vi "phan_songsong.vi"() -> ()   [LabVIEW 2019]
uses:
  <vilib>/Platform/TimedLoop/XDataNode/timing_clust.ctl
  <vilib>/Platform/TimedLoop/XDataNode/nitl_modes.ctl
  <vilib>/Platform/TimedLoop/XDataNode/wakeup.ctl
  <vilib>/platform/TimedLoop/XDataNode/XDataNode.xnode
  <vilib>/Platform/TimedLoop/XDataNode/XDNodeRunTimeDep.lvlib
  <vilib>/ptbypt/NI_PtbyPt.lvlib
panel:
  out "S":dbl
  out "yo":dbl
  out "xo":dbl
  out "yb":dbl
  out "xb":dbl
  out "ya":dbl
  out "xa":dbl
  out "c":dbl
  out "y_o":dbl
  out "x_o":dbl
  in  "vantocgocmax":dbl=1.5
  in  "vantocmax":dbl=0.5
  out "phi_ph":dbl
  out "wdk":dbl
  out "phi_sp":dbl
  in  "Kiw":dbl
  in  "Kpw":dbl=3.0
  in  "Kdw":dbl
  out "Vxdk":dbl
  out "Vydk":dbl
  in  "Kdv3":dbl
  in  "Kiv3":dbl=28.5
  in  "Kpv3":dbl=0.7
  in  "Kdv2":dbl
  in  "Kiv2":dbl=28.5
  in  "Kpv2":dbl=0.7
  out "Ts":dbl=10.0
  out "TOA DO 2":dbl[][](array[numeric])
  out "sailechxy":cluster{"e_phi":dbl, "e_x":dbl, "e_y":dbl}(graph)
  in  "Kdxy":dbl
  in  "Kixy":dbl
  in  "Kpxy":dbl=4.0
  in  "?":enum32{"DUONG 2", "DUONGTRON", "NHAP DIEM"}(tab)
  in  "xstart":dbl format="%#_13g"
  in  "xend":dbl=2.0
  in  "time2":dbl=10.0
  in  "R":dbl=0.6
  in  "phi_end":dbl=15.71
  in  "phi_start":dbl=3.14159 format="%#_13g"
  out "time":dbl
  in  "y2":dbl
  in  "x1":dbl
  in  "x2":dbl
  in  "x3":dbl
  in  "y3":dbl
  in  "y1":dbl
  in  "x4":dbl
  in  "y4":dbl
  out "time":dbl
  out "buoc":dbl
  out "V_ph":dbl
  out "w_ph3":dbl
  out "w_ph2":dbl
  out "w_ph1":dbl
  in  "RESETMAP":bool=TRUE caption="Reset"
  out "duty3":dbl
  out "duty2":dbl
  out "duty1":dbl
  in  "RESET":bool
  out "Y_sp":dbl
  out "X_sp":dbl
  out "Y_ph":dbl
  out "X_ph":dbl
  out "Map":cluster{"Y":dbl[], "Y":dbl[]}[](graph)
  out "V3_sp":dbl
  out "V3_ph":dbl
  out "VAN TOC":T1(graph)
  in  "Kdv1":dbl
  in  "Kiv1":dbl=28.5
  in  "Kpv1":dbl=0.7
  out "V2_ph":dbl
  out "V1_ph":dbl
  out "V2_sp":dbl
  out "V1_sp":dbl
  in  "START":bool
  # "HE THONG"
  # "PID VI TRI"
  # "PID TOC DO"
  # "VI TRI DIEU KHIEN\n(m)"
  # "VI TRI PHAN HOI\n(m)"
  # "Van toc dat"
  # "VAN TOC DIEU KHIEN\n(m/s)"
  # "VAN TOC PHAN HOI\n(m/s)"
  # "DUTY"
  # "TOC DO PHAN HOI (rad/s)"
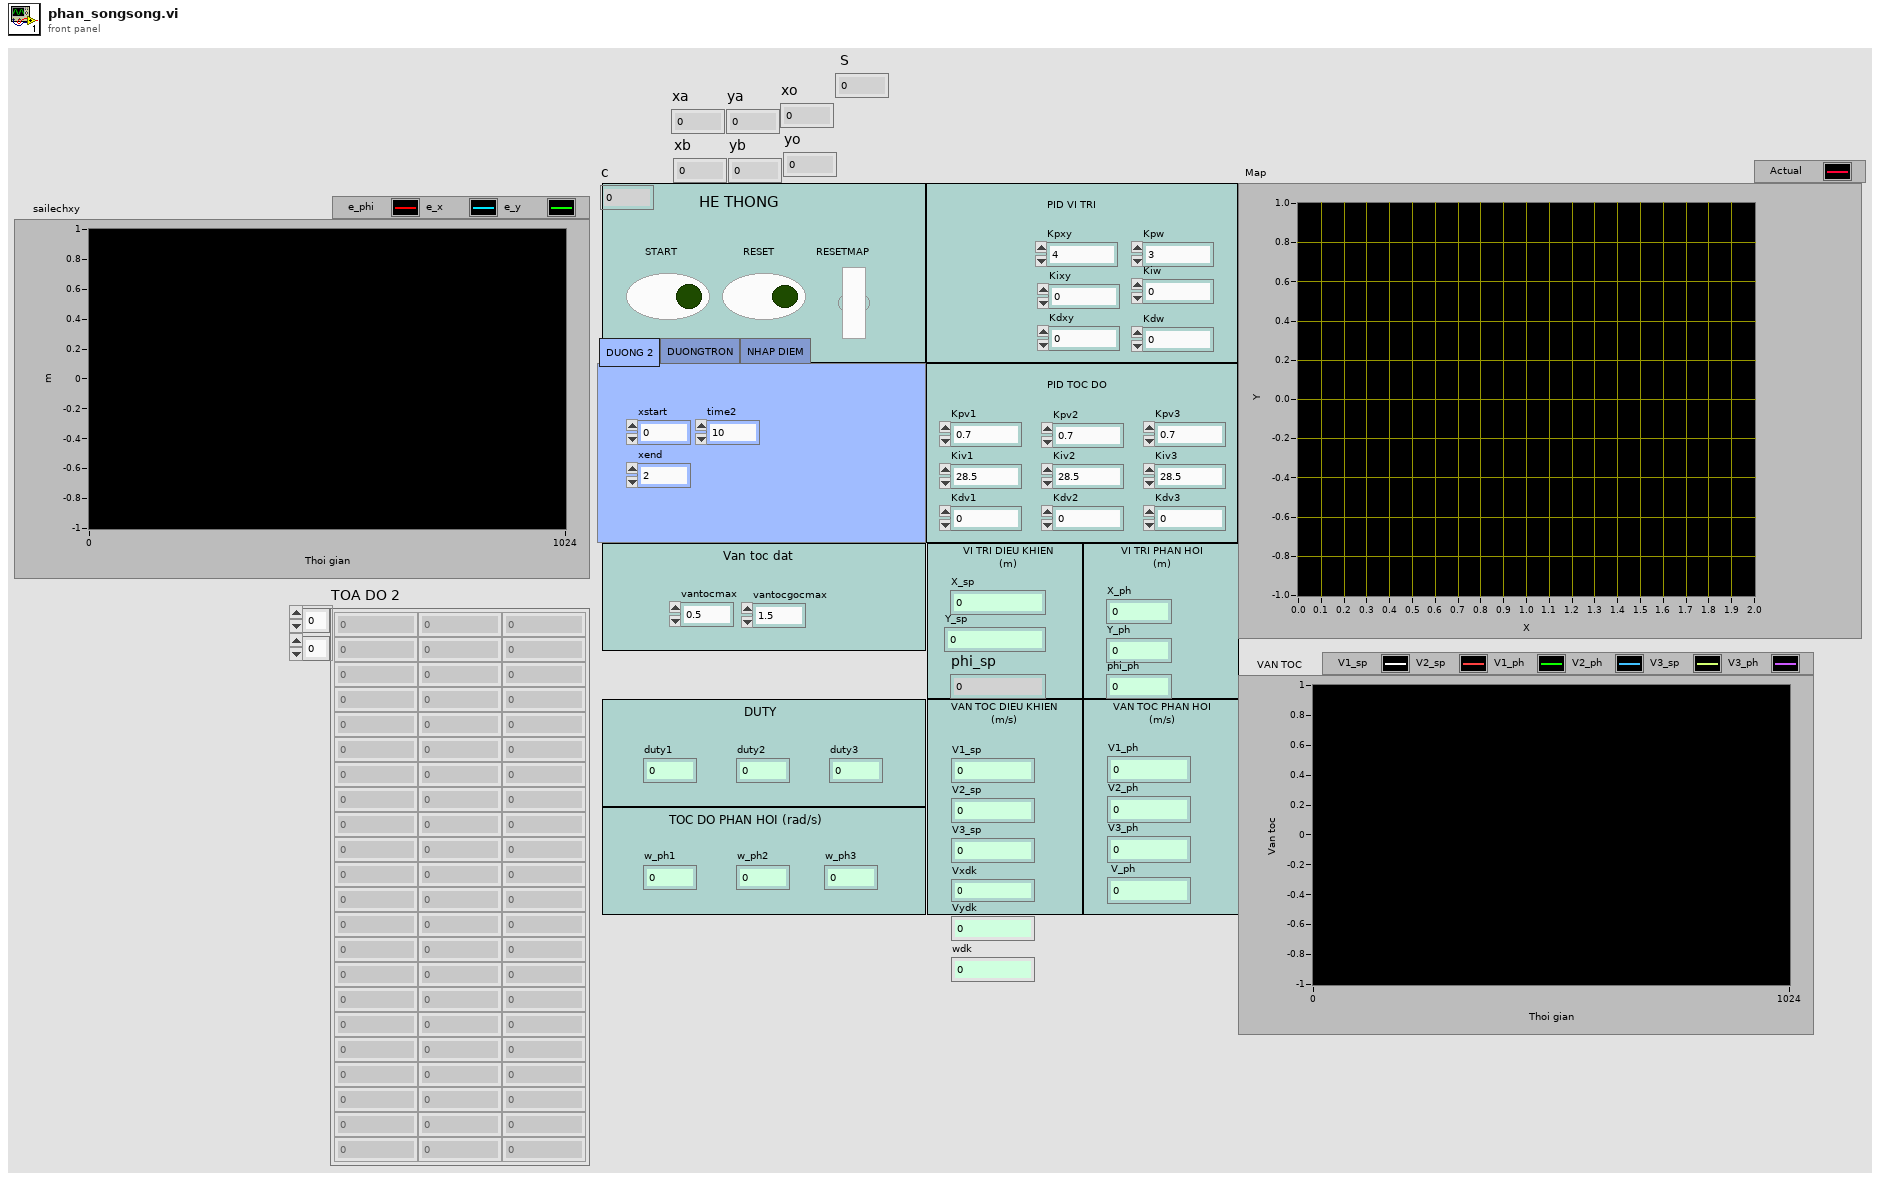
[diagram p1: front panel]
types:
  T1 = cluster{dbl, dbl, "V1_ph":dbl, "V2_ph":dbl, dbl, "V3_ph":dbl}
  T2 = typedef "XDNodeRunTimeDep.lvlib/timing_clust.ctl" = cluster{"Expected End [f-1]":u64, "Actual End [f-1]":u64, "Finished Late? [f-1]":bool, "Expected End [i-1]":u64, "Actual End [i-1]":u64, "Finished Late? [i-1]":bool, "Expected Start [i]":u64, "Actual Start [i]":u64, "Expected Start [f]":u64, "Actual Start [f]":u64, "Source Name":string, "Structure Name":string, "Period":i64, "Deadline":i64, "Offset":i64, "Start":i64, "Priority":i32, "Timeout":i32, "Mode":T3, "Wakeup Reason":T4, "Error":errorcluster, "Source Type":string, "Secondary Source Type":string, "Global End Time":u64, "Global Start Time":u64, "Frame Duration":u64, "Iteration Duration":u64, "Assigned CPU":i32, "I/O Scan Engine Mode":u32}
  T3 = typedef "XDNodeRunTimeDep.lvlib/nitl_modes.ctl" = enum32{"No Change", "Process missed periods, maintain original phase", "Discard missed periods, maintain original phase", "Process missed periods, ignore original phase", "Discard missed periods, ignore original phase"}
  T4 = typedef "XDNodeRunTimeDep.lvlib/wakeup.ctl" = enum32{"Normal", "Aborted", "Asynchronous wakeup", "Timing source error", "Timed loop error", "Timeout"}
  T5 = cluster{"V1_sp":dbl, "V_ph1":dbl, "V2_sp":dbl, "V_ph2":dbl, "V3_sp":dbl, "V_ph3":dbl}
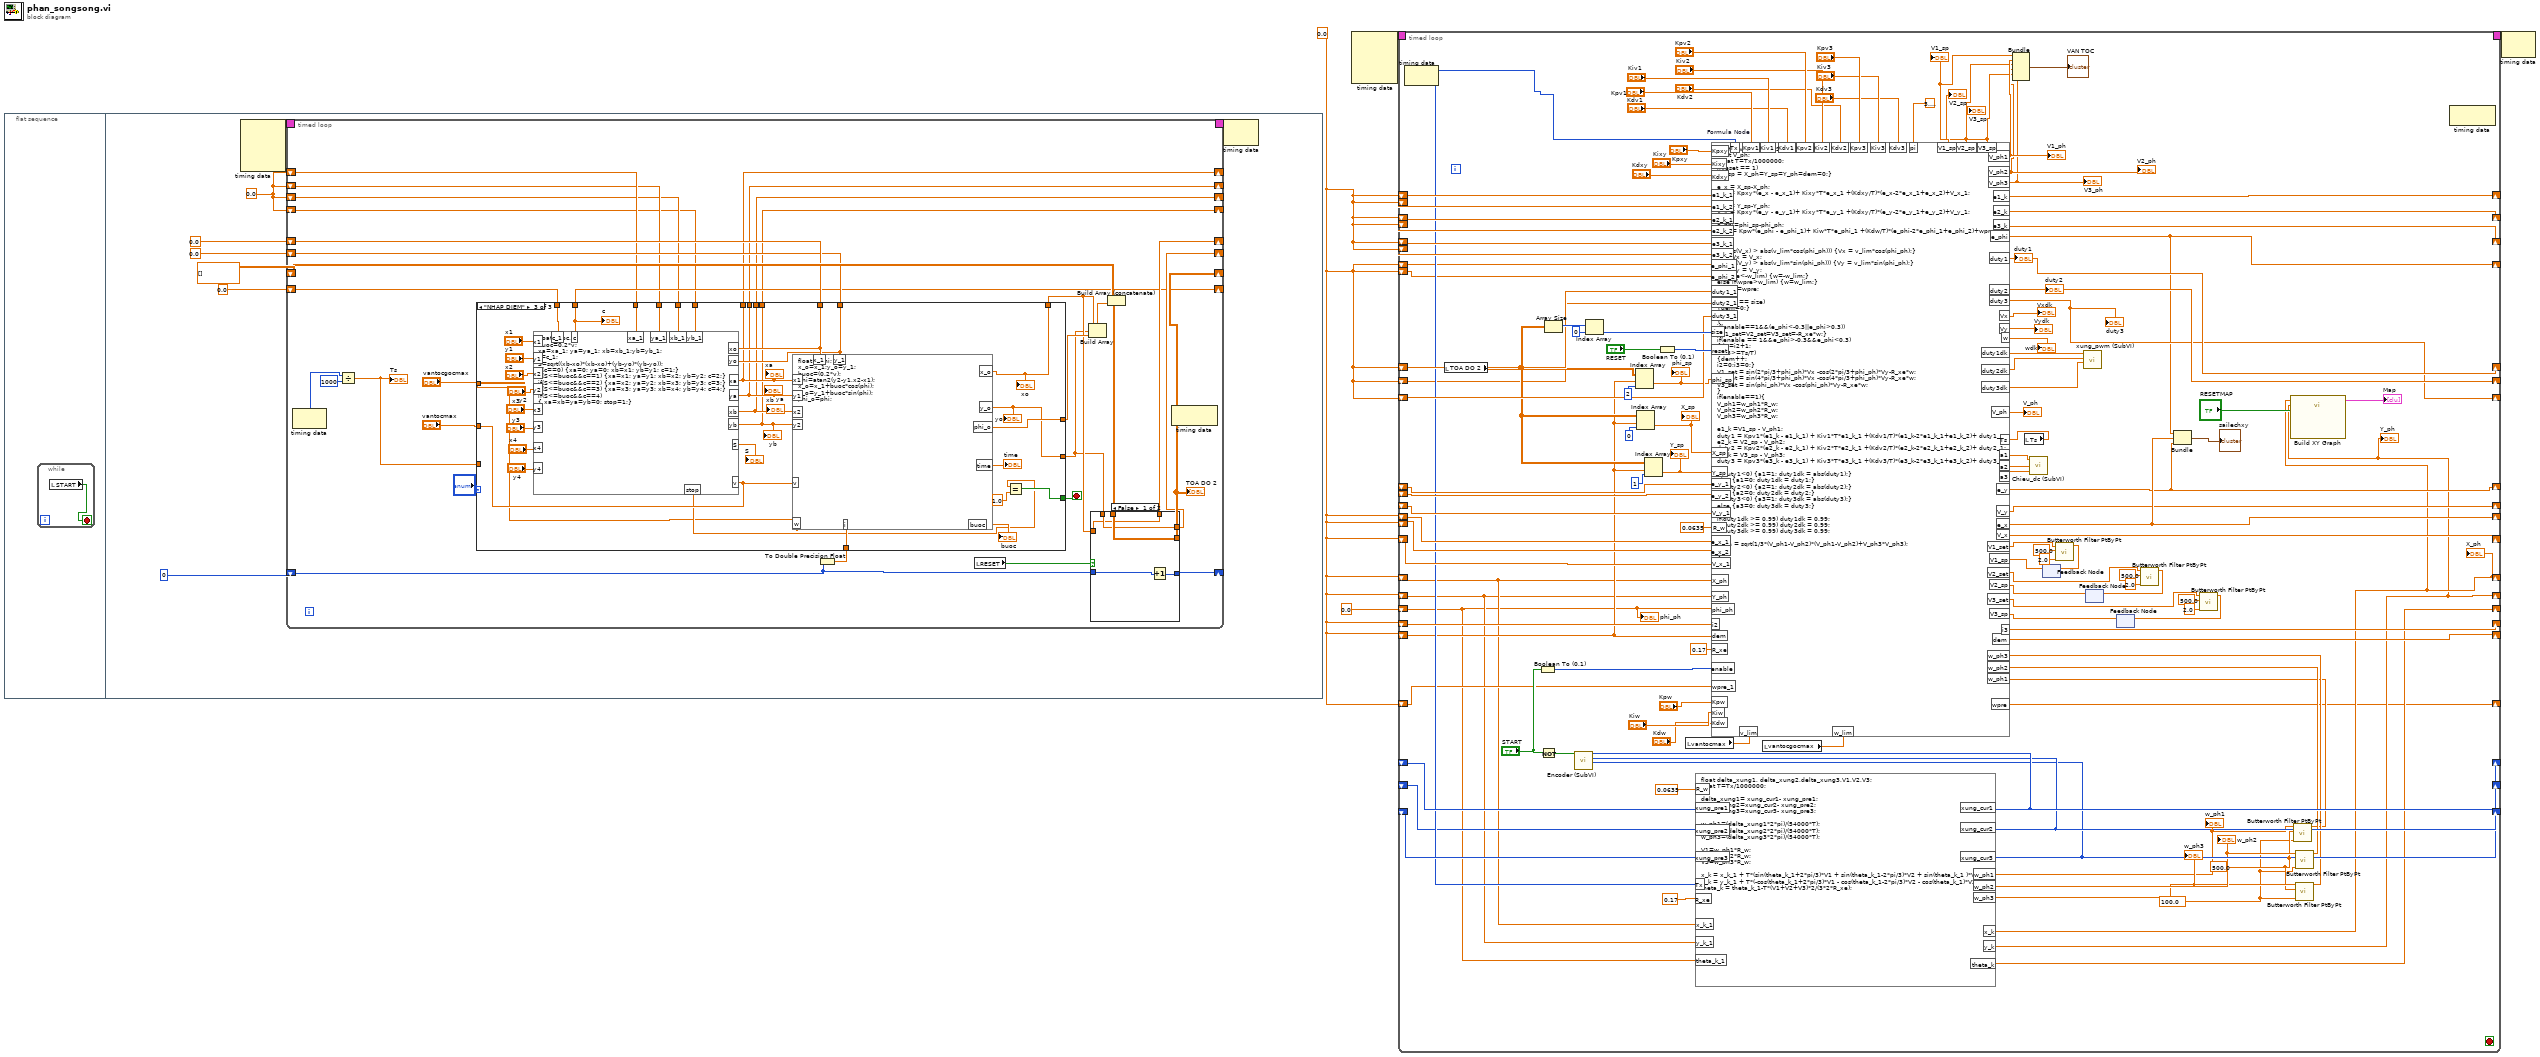
[diagram p0: block diagram]
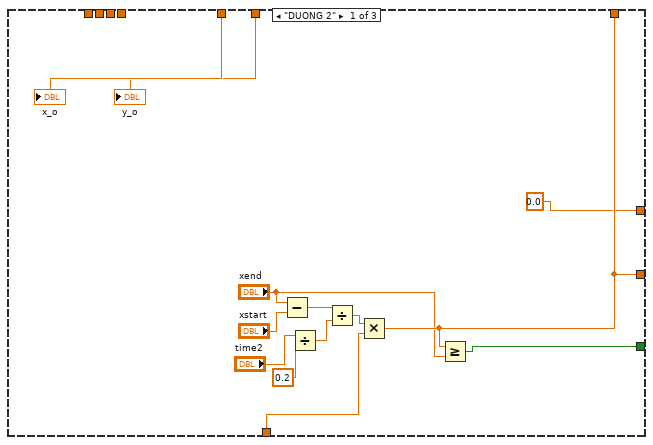
[diagram p2: hidden frame]
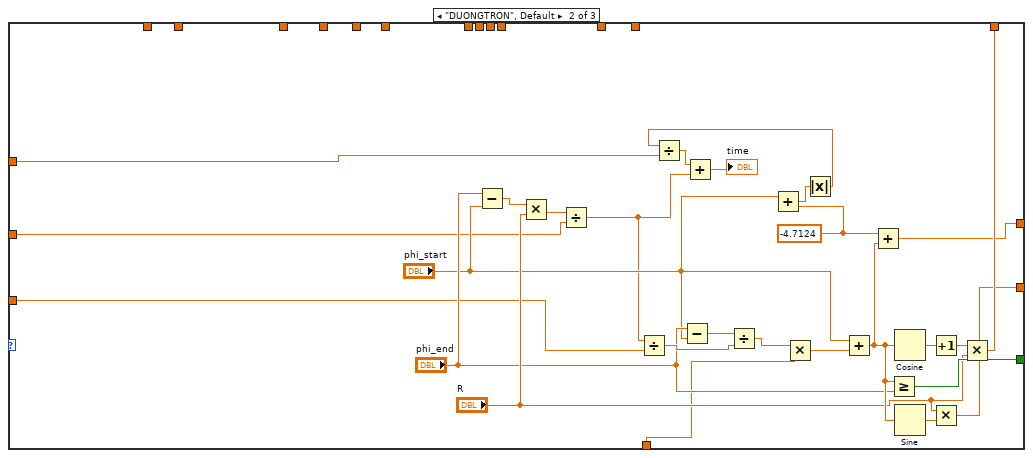
[diagram p3: hidden frame]
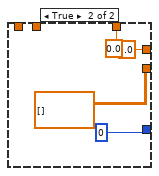
[diagram p4: hidden frame]
diagram:
  w2 = 0.0 ("e1")
  n1 = flat-sequence {
    frame #0 {
      n2 = while {
        stop <- w5 stop-if-true
        n3 = local read "START"() -> (w5:bool)
      }
    }
    frame #1 {
      w6 = 0.0 ("xa")
      n4 = node-c288() -> (w13:T2)  [unwired: 4 in]
      n5 = timed-loop {
        timing: w13 -> [_]
        timing-out: [_] -> w12
        shift-right: [w39] -> _
        shift-left: dbl[][] [] -> [w43]
        shift-right: [w41] -> _
        shift-left: 0 -> [w40]
        shift-right: [w25] -> _
        shift-left: 0.0 ("y_o") -> [w29]
        shift-right: [w26] -> _
        shift-left: 0.0 ("x_o") -> [w30]
        shift-right: [w23] -> _
        shift-left: 0.0 ("c") -> [w24]
        shift-right: [w17] -> _
        shift-left: w6 -> [w21]
        shift-right: [w16] -> _
        shift-left: w6 -> [w20]
        shift-right: [w15] -> _
        shift-left: w6 -> [w19]
        shift-right: [w14] -> _
        shift-left: w6 -> [w18]
        stop <- w36 stop-if-true
        n6 = node-c288() -> (w38:i64)  [unwired: 1 in]
        n7 = Divide(x=w38, y=i64 1000) -> (x/y=w22:dbl)
        "Ts" <- w22
        n8 = To Double Precision Float(number=w40) -> (double precision float=w45:dbl)
        n9 = case shown="\"NHAP DIEM\"" "?" {
          tunnel: w45 -> [w55 w62 w117]
          tunnel: [w54 w81 w96] -> w28
          tunnel: [w54 w80 w95] -> w27
          tunnel: [w52 w79 w115] -> w36
          tunnel: [0.0 w74 w114] -> w33
          tunnel: "vantocmax" -> [_ w61 w101]
          tunnel: "vantocgocmax" -> [_ w60 w97]
          tunnel: w30 -> [w47 _ w99]
          tunnel: w29 -> [w46 _ w98]
          tunnel: w24 -> [_ _ w103]
          tunnel: [_ _ w102] -> w23
          tunnel: w22 -> [_ w59 _]
          tunnel: w21 -> [_ _ w94]
          tunnel: w20 -> [_ _ w93]
          tunnel: w19 -> [_ _ w92]
          tunnel: w18 -> [_ _ w91]
          tunnel: [_ _ w90] -> w17
          tunnel: [_ _ w89] -> w16
          tunnel: [_ _ w88] -> w15
          tunnel: [_ _ w87] -> w14
          frame "DUONG 2" {
            n10 = Subtract(x="xend", y="xstart") -> (x-y=w57:dbl)
            n11 = Divide(x="time2", y=0.2) -> (x/y=w49:dbl)
            n12 = Divide(x=w57, y=w49) -> (x/y=w56:dbl)
            n13 = Multiply(x=w56, y=w55) -> (x*y=w54:dbl)
            n14 = Greater Or Equal?(x=w54, y="xend") -> (x >= y?=w52:bool)
            "x_o" <- w47
            "y_o" <- w46
          }
          frame "DUONGTRON", Default {
            w69 = -4.7124 ("x")
            n15 = Subtract(x="phi_end", y="phi_start") -> (x-y=w70:dbl)
            n16 = Multiply(x=w70, y="R") -> (x*y=w72:dbl)
            n17 = Divide(x=w72, y=w61) -> (x/y=w64:dbl)
            n18 = Divide(x=w64, y=w59) -> (x/y=w76:dbl)
            n19 = Subtract(x="phi_end", y="phi_start") -> (x-y=w78:dbl)
            n20 = Divide(x=w78, y=w76) -> (x/y=w77:dbl)
            n21 = Add(x="phi_start", y=w69) -> (x+y=w67:dbl)
            n22 = Multiply(x=w77, y=w62) -> (x*y=w85:dbl)
            n23 = Absolute Value(x=w67) -> (abs(x)=w66:dbl)
            n24 = Divide(x=w66, y=w60) -> (x/y=w65:dbl)
            n25 = Add(x=w65, y=w64) -> (x+y=→"time":dbl)
            n26 = Add(x="phi_start", y=w85) -> (x+y=w75:dbl)
            n27 = Add(x=w69, y=w75) -> (x+y=w74:dbl)
            n28 = Greater Or Equal?(x=w75, y="phi_end") -> (x >= y?=w79:bool)
            n29 = Cosine(x=w75) -> (cos(x)=w84:dbl)
            n30 = Sine(x=w75) -> (sin(x)=w82:dbl)
            n31 = Increment(x=w84) -> (x+1=w83:dbl)
            n32 = Multiply(x="R", y=w82) -> (x*y=w80:dbl)
            n33 = Multiply(x=w83, y="R") -> (x*y=w81:dbl)
          }
          frame "NHAP DIEM" {
            n34 = formula code="float buoc,S;\nbuoc=0.2*v;\nxa=xa_1; ya=ya_1; xb=xb_1;yb=yb_1;\nc=c_1;\nS=sqrt((xb-xo)*(xb-xo)+(yb-yo)*(yb-yo));\nif(c==0) {xa=0; ya=0; xb=x1; yb=y1; c=1;}\nif(S<=buoc&&c==1) {xa=x1; ya=y1; xb=x2; yb=y2; c=2;}\nif(S<=buoc&&c==2) {xa=x2; ya=y2; xb=x3; yb=y3; c=3;}\nif(S<=buoc&&c==3) {xa=x3; ya=y3; xb=x4; yb=y4; c=4;}\nif(S<=buoc&&c==4) \n{ xa=xb=ya=yb=0; stop=1;}"("x1"="x1", "y1"="y1", "x2"="x2", "y2"="y2", "x3"="x3", "y3"="y3", "x4"="x4", "y4"="y4", "c_1"=w103, "xo"=w99, "yo"=w98, "v"=w101, "xa_1"=w94, "ya_1"=w93, "xb_1"=w92, "yb_1"=w91) -> ("xa"=w90:dbl, "ya"=w89:dbl, "xb"=w88:dbl, "yb"=w87:dbl, "c"=w102:dbl, "stop"=w100:dbl, "S"=→"S":dbl)
            "c" <- w102
            "xa" <- w90
            "ya" <- w89
            "xb" <- w88
            "yb" <- w87
            n35 = formula code="float S,phi;\nx_o=x_1;y_o=y_1;\nbuoc=(0.2*v);\nphi=atan2(y2-y1,x2-x1);\nx_o=x_1+buoc*cos(phi);\ny_o=y_1+buoc*sin(phi);\nphi_o=phi;"("i"=w117, "x1"=w90, "y1"=w89, "v"=w101, "w"=w97, "x_1"=w99, "y_1"=w98, "x2"=w88, "y2"=w87) -> ("x_o"=w96:dbl, "y_o"=w95:dbl, "phi_o"=w114:dbl, "time"=→"time":dbl, "buoc"=→"buoc":dbl)
            "xo" <- w96
            "yo" <- w95
            n36 = Equal?(x=w100, y=1.0) -> (x = y?=w115:bool)
          }
        }
        n37 = local read "RESET"() -> (w35:bool)
        n38 = Build Array(w28, w27, w33) -> (w44:dbl[])
        n39 = Build Array (concatenate)(w43, w44) -> (w42:dbl[][])
        n40 = case shown="False" w35 {
          tunnel: w42 -> [w122 _]
          tunnel: [w122 dbl[][] []] -> w39
          tunnel: [w121 0] -> w41
          tunnel: w40 -> [w120 _]
          tunnel: w28 -> [w118 _]
          tunnel: w27 -> [w119 _]
          tunnel: [w118 0.0 ("x_o")] -> w26
          tunnel: [w119 0.0 ("y_o")] -> w25
          frame False {
            n41 = Increment(x=w120) -> (x+1=w121:i32)
          }
          frame True {
          }
        }
        "TOA DO 2" <- w39
        n42 = node-c288() -> ()  [unwired: 1 in, 1 out]
      }
      n43 = node-c288(w12) -> ()  [unwired: 1 out]
    }
  }
  n44 = node-c288() -> (w4:T2)  [unwired: 4 in]
  n45 = timed-loop {
    timing: w4 -> [_]
    timing-out: [_] -> w3
    shift-right: [w259] -> _
    shift-left: w2 -> [w257]
    shift-right: [w258] -> _
    shift-left: w2 -> [w216]
    shift-right: [w250] -> _
    shift-left: w2 -> [w249]
    shift-right: [w145] -> _
    shift-left: w2 -> [w142]
    shift-right: [w144] -> _
    shift-left: w2 -> [w141]
    shift-right: [w248] -> _
    shift-left: w2 -> [w156]
    shift-right: [w228] -> _
    shift-left: w2 -> [w229]
    shift-right: [w227] -> _
    shift-left: w2 -> [w225]
    shift-right: [w226] -> _
    shift-left: w2 -> [w153]
    shift-right: [w154] -> _
    shift-left: w2 -> [w224]
    shift-right: [w219] -> _
    shift-left: _ -> [w221]
    shift-right: [w218] -> _
    shift-left: _ -> [w150]
    shift-right: [w217] -> _
    shift-left: _ -> [w220]
    shift-right: [w169] -> _
    shift-left: w2 -> [w211]
    shift-right: [w209] -> _
    shift-left: w2 -> [w210]
    shift-left: w2 -> [w205]
    shift-left: w2 -> [w204]
    shift-left: w2 -> [w203]
    shift-left: w2 -> [w202]
    shift-right: [w160] -> _
    shift-left: _ -> [w165]
    shift-right: [w167] -> _
    shift-left: _ -> [w166]
    shift-left: _ -> [w164]
    shift-right: [w143] -> _
    shift-left: 0.0 ("phi_ph") -> [w135]
    shift-right: [w138] -> _
    shift-left: w2 -> [w152]
    shift-left: w2 -> [w151]
    shift-right: [w134] -> _
    shift-left: w2 -> [w149]
    stop <- _ stop-if-true
    w196 = 100.0 ("flw")
    w197 = 500.0 ("sampling freq: fs")
    n46 = node-c288() -> (w159:i64)  [unwired: 1 in]
    n47 = local read "TOA DO 2"() -> (w157:dbl[][])
    n48 = Boolean To (0,1)(Boolean="START") -> (0, 1=w256:i16)
    n49 = Not(x="START") -> (.not. x?=w231:bool)
    n50 = Array Size(array=w157) -> (size(s)=w244:i32[])
    n51 = call "Encoder (SubVI).vi"("Boolean"=w231) -> ("Counter Value3"=w217:i32, "Counter Value 2"=w218:i32, "Counter Value"=w219:i32)  [unwired: 8 in]
    n52 = Index Array(array=w244, index=0) -> (element=w242:i32)
    n53 = Index Array(array=w157, index (row)=w156, index (col)=2 ("disabled index (col)")) -> (element=w155:dbl)
    "phi_sp" <- w155
    n54 = Index Array(array=w157, index (row)=w156, index (col)=0 ("disabled index (col)")) -> (element=w246:dbl)
    "X_sp" <- w246
    n55 = Index Array(array=w157, index (row)=w156, index (col)=1 ("disabled index (col)")) -> (element=w245:dbl)
    "Y_sp" <- w245
    n56 = Boolean To (0,1)(Boolean="RESET") -> (0, 1=w241:i16)
    n57 = local read "vantocmax"() -> (w133:dbl)
    n58 = formula code="float delta_xung1, delta_xung2,delta_xung3,V1,V2,V3;\nfloat T=Tx/1000000;\n\ndelta_xung1= xung_cur1- xung_pre1;\ndelta_xung2=xung_cur2- xung_pre2;\ndelta_xung3=xung_cur3- xung_pre3; \n\nw_ph1=(delta_xung1*2*pi)/(54000*T);\nw_ph2=(delta_xung2*2*pi)/(54000*T);\nw_ph3=(delta_xung3*2*pi)/(54000*T);\n\nV1=w_ph1*R_w;\nV2=w_ph2*R_w;\nV3=w_ph3*R_w;\n\nx_k = x_k_1 + T*(sin(theta_k_1+2*pi/3)*V1 + sin(theta_k_1-2*pi/3)*V2 + sin(theta_k_1 )*V3)*2/3;\ny_k = y_k_1 + T*(-cos(theta_k_1+2*pi/3)*V1 - cos(theta_k_1-2*pi/3)*V2 - cos(theta_k_1)*V3)*2/3;\ntheta_k = theta_k_1-T*(V1+V2+V3)*2/(3*2*R_xe);"("xung_pre1"=w221, "xung_pre2"=w150, "xung_pre3"=w220, "xung_cur1"=w219, "xung_cur2"=w218, "xung_cur3"=w217, "Tx"=w159, "x_k_1"=w142, "y_k_1"=w141, "theta_k_1"=w135, "R_w"=0.0635 ("input variable"), "R_xe"=0.17 ("input variable")) -> ("w_ph1"=w187:dbl, "w_ph2"=w199:dbl, "w_ph3"=w198:dbl, "x_k"=w145:dbl, "y_k"=w144:dbl, "theta_k"=w143:dbl)
    "X_ph" <- w145
    "Y_ph" <- w144
    "w_ph1" <- w187
    "w_ph2" <- w199
    "w_ph3" <- w198
    n59 = local read "vantocgocmax"() -> (w132:dbl)
    n60 = local read "Ts"() -> (w161:dbl)
    n61 = feedback #1() -> (w177:dbl)  [unwired: 1 in]
    n62 = feedback #2() -> (w174:dbl)  [unwired: 1 in]
    n63 = feedback #3() -> (w171:dbl)  [unwired: 1 in]
    n64 = call "Build XY Graph"("Reset"="RESETMAP", "Y Input"=w144, "X Input"=w145) -> ("XY Graph"=→"Map":cluster{"X":dbl[], "Y":dbl[]}[])  [unwired: 7 in, 1 out]
    n65 = call <vilib>:"Butterworth Filter PtByPt.vi"("low cutoff freq: fl"=w196, "sampling freq: fs"=w197, "x"=w187) -> ("Filtered x"=w186:dbl)  [unwired: 6 in, 1 out]
    n66 = call <vilib>:"Butterworth Filter PtByPt.vi"("low cutoff freq: fl"=w196, "sampling freq: fs"=w197, "x"=w199) -> ("Filtered x"=w195:dbl)  [unwired: 6 in, 1 out]
    n67 = call <vilib>:"Butterworth Filter PtByPt.vi"("low cutoff freq: fl"=w196, "sampling freq: fs"=w197, "x"=w198) -> ("Filtered x"=w194:dbl)  [unwired: 6 in, 1 out]
    n68 = formula code="float V,Vtest, S_sp, S_ph, Vx, Vy,w;\nfloat V_ph;\n float T=Tx/1000000;\nif(reset == 1)\n{X_sp = X_ph=Y_sp=Y_ph=dem=0;}\n\ne_x = X_sp-X_ph; \nV_x = Kpxy*(e_x - e_x_1)+ Kixy*T*e_x_1 +(Kdxy/T)*(e_x-2*e_x_1+e_x_2)+V_x_1;\n\ne_y = Y_sp-Y_ph; \nV_y = Kpxy*(e_y - e_y_1)+ Kixy*T*e_y_1 +(Kdxy/T)*(e_y-2*e_y_1+e_y_2)+V_y_1;\n\ne_phi=phi_sp-phi_ph;\nwpre= Kpw*(e_phi - e_phi_1)+ Kiw*T*e_phi_1 +(Kdw/T)*(e_phi-2*e_phi_1+e_phi_2)+wpre_1;\n\n\nif (abs(V_x) > abs(v_lim*cos(phi_ph))) {Vx = v_lim*cos(phi_ph);} \nelse Vx = V_x;\nif (abs(V_y) > abs(v_lim*sin(phi_ph))) {Vy = v_lim*sin(phi_ph);} \nelse Vy = V_y;\nif (wpre<-w_lim) {w=-w_lim;}\nelse if(wpre>w_lim) {w=w_lim;}\nelse w=wpre;\n\nif(dem == size)\n{dem=0;}\nelse\n{ \nif(enable==1&&(e_phi<-0.3||e_phi>0.3))\n{V1_set=V2_set=V3_set=-R_xe*w;}\nif(enable == 1&&e_phi>-0.3&&e_phi<0.3)\n{ i3=i2+1;\nif (i3>=Ts/T)\n{dem++;\ni2=0;i3=0;}\nV1_set = sin(2*pi/3+phi_ph)*Vx -cos(2*pi/3+phi_ph)*Vy-R_xe*w;\nV2_set = sin(4*pi/3+phi_ph)*Vx -cos(4*pi/3+phi_ph)*Vy-R_xe*w;\nV3_set = sin(phi_ph)*Vx -cos(phi_ph)*Vy-R_xe*w;\n}\nif(enable==1){\nV_ph1=w_ph1*R_w;\nV_ph2=w_ph2*R_w;\nV_ph3=w_ph3*R_w;\n\ne1_k =V1_sp - V_ph1;\nduty1 = Kpv1*(e1_k - e1_k_1) + Kiv1*T*e1_k_1 +(Kdv1/T)*(e1_k-2*e1_k_1+e1_k_2)+ duty1_1;\ne2_k = V2_sp - V_ph2;\nduty2 = Kpv2*(e2_k - e2_k_1) + Kiv2*T*e2_k_1 +(Kdv2/T)*(e2_k-2*e2_k_1+e2_k_2)+ duty2_1;\ne3_k = V3_sp - V_ph3;\nduty3 = Kpv3*(e3_k - e3_k_1) + Kiv3*T*e3_k_1 +(Kdv3/T)*(e3_k-2*e3_k_1+e3_k_2)+ duty3_1;\n\nif(duty1<0) {a1=1; duty1dk = abs(duty1);}\nelse {a1=0; duty1dk = duty1;}\nif(duty2<0) {a2=1; duty2dk = abs(duty2);}\nelse {a2=0; duty2dk = duty2;}\nif(duty3<0) {a3=1; duty3dk = abs(duty3);}\nelse {a3=0; duty3dk = duty3;}\n\nif(duty1dk >= 0.99) duty1dk = 0.99;\nif(duty2dk >= 0.99) duty2dk = 0.99;\nif(duty3dk >= 0.99) duty3dk = 0.99;\n\nV_ph = sqrt(1/3*(V_ph1-V_ph2)*(V_ph1-V_ph2)+V_ph3*V_ph3);\n\n}\n}"("Kpv1"="Kpv1", "Kiv1"="Kiv1", "Kdv1"="Kdv1", "pi"=3.141592653589793, "e1_k_1"=w257, "e2_k_1"=w216, "enable"=w256, "Tx"=w159, "e3_k_1"=w249, "X_ph"=w142, "X_sp"=w246, "Y_sp"=w245, "Y_ph"=w141, "dem"=w156, "size"=w242, "reset"=w241, "i2"=w229, "duty1_1"=w225, "duty2_1"=w153, "duty3_1"=w224, "w_ph1"=w186, "w_ph2"=w195, "w_ph3"=w194, "e_x_1"=w211, "V_x_1"=w210, "Kpxy"="Kpxy", "Kixy"="Kixy", "Kdxy"="Kdxy", "e1_k_2"=w205, "e2_k_2"=w204, "e3_k_2"=w203, "e_x_2"=w202, "Ts"=w161, "Kpv2"="Kpv2", "Kiv2"="Kiv2", "Kdv2"="Kdv2", "Kpv3"="Kpv3", "Kiv3"="Kiv3", "Kdv3"="Kdv3", "V1_sp"=w177, "V2_sp"=w174, "V3_sp"=w171, "R_w"=0.0635 ("input variable"), "e_y_1"=w165, "e_y_2"=w164, "V_y_1"=w166, "phi_sp"=w155, "phi_ph"=w135, "e_phi_1"=w152, "e_phi_2"=w151, "wpre_1"=w149, "Kpw"="Kpw", "Kiw"="Kiw", "Kdw"="Kdw", "R_xe"=0.17 ("input variable"), "v_lim"=w133, "w_lim"=w132) -> ("V1_sp"=w239:dbl, "V_ph1"=w238:dbl, "V_ph2"=w236:dbl, "e1_k"=w259:dbl, "e2_k"=w258:dbl, "V2_sp"=w237:dbl, "duty1"=w227:dbl, "duty2"=w226:dbl, "e3_k"=w250:dbl, "V_ph3"=w235:dbl, "V3_sp"=w234:dbl, "duty3"=w154:dbl, "a1"=w230:dbl, "a2"=w223:dbl, "a3"=w222:dbl, "dem"=w248:dbl, "i3"=w228:dbl, "duty1dk"=w215:dbl, "duty2dk"=w214:dbl, "duty3dk"=w213:dbl, "V_ph"=→"V_ph":dbl, "e_x"=w169:dbl, "V_x"=w209:dbl, "V1_set"=w179:dbl, "V2_set"=w176:dbl, "V3_set"=w173:dbl, "e_y"=w160:dbl, "V_y"=w167:dbl, "Vx"=→"Vxdk":dbl, "Vy"=→"Vydk":dbl, "e_phi"=w138:dbl, "wpre"=w134:dbl, "w"=→"wdk":dbl)
    "V1_sp" <- w239
    "V2_sp" <- w237
    "V1_ph" <- w238
    "V2_ph" <- w236
    "V3_ph" <- w235
    "V3_sp" <- w234
    "duty1" <- w227
    "duty2" <- w226
    "duty3" <- w154
    n69 = Bundle("V1_sp"=w239, "V_ph1"=w238, "V2_sp"=w237, "V_ph2"=w236, "V3_sp"=w234, "V_ph3"=w235) -> (→"VAN TOC":T5)  [unwired: 1 in]
    n70 = call "Chieu_dc (SubVI).vi"("a3"=w222, "a2"=w223, "a1"=w230) -> ()
    n71 = call <vilib>:"Butterworth Filter PtByPt.vi"("low cutoff freq: fl"=2.0, "sampling freq: fs"=500.0, "x"=w179) -> ("Filtered x"=w178:dbl)  [unwired: 6 in, 1 out]
    n72 = feedback-in #1(w178) -> ()
    n73 = call "xung_pwm (SubVI).vi"("duty3 in"=w213, "duty2 in"=w214, "duty1 in"=w215) -> ()  [unwired: 6 in, 3 out]
    n74 = call <vilib>:"Butterworth Filter PtByPt.vi"("low cutoff freq: fl"=2.0, "sampling freq: fs"=500.0, "x"=w176) -> ("Filtered x"=w175:dbl)  [unwired: 6 in, 1 out]
    n75 = feedback-in #2(w175) -> ()
    n76 = Bundle("e_phi"=w138, "e_x"=w169, "e_y"=w160) -> (→"sailechxy":cluster{"e_phi":dbl, "e_x":dbl, "e_y":dbl})  [unwired: 1 in]
    n77 = call <vilib>:"Butterworth Filter PtByPt.vi"("low cutoff freq: fl"=2.0, "sampling freq: fs"=500.0, "x"=w173) -> ("Filtered x"=w172:dbl)  [unwired: 6 in, 1 out]
    n78 = feedback-in #3(w172) -> ()
    n79 = node-c288() -> ()  [unwired: 1 in, 1 out]
    "phi_ph" <- w135
  }
  n80 = node-c288(w3) -> ()  [unwired: 1 out]
